vi "Build Array Name.vi"(8 "Name In":string, 9 "Array":u32[](array[numeric]), 10 "Iteration":i32, 11 "Iterations":i32) -> (0 "Name Out":string)   [LabVIEW 2012]
doc: "This VI was created for use with the Read/Write Cluster VIs. It builds the name used as the INI key for arrays which includes the array dimensions.\n\nFreeware from Moore Good Ideas, www.mooregoodideas.com. Do not remove this line."
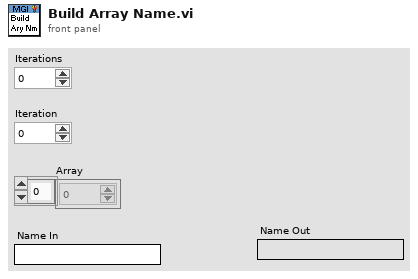
[diagram p1: front panel]
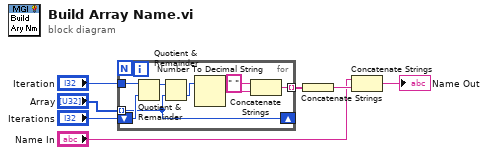
[diagram p0: block diagram]
diagram:
  n1 = for {
    tunnel: [w14] -> w4 mode=indexing
    tunnel: "Iteration" -> [w12]
    tunnel: "Array" -> [w9] mode=indexing
    shift-right: [w9] -> _
    shift-left: "Iterations" -> [w11]
    n2 = Quotient & Remainder(x=w12, y=w11) -> (x-y*floor(x/y)=w13:u32)  [unwired: 1 out]
    n3 = Quotient & Remainder(x=w13, y=w9) -> (floor(x/y)=w10:u32)  [unwired: 1 out]
    n4 = Number To Decimal String(number=w10) -> (decimal integer string=w15:string)  [unwired: 1 in]
    n5 = Concatenate Strings(" " ("string"), w15) -> (w14:string)
  }
  n6 = Concatenate Strings(w4) -> (w2:string)
  n7 = Concatenate Strings("Name In", w2) -> (→"Name Out":string)
